vi "ResetKnob.vi"(1 "name":string, 2 "camera":u64, 3 "knobRef":refnum<vi>) -> ()   [LabVIEW 2019]
uses:
  EmergentCameraC/EmergentCameraC.lvlib
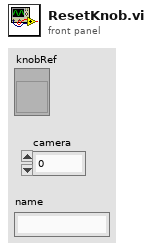
[diagram p1: front panel]
types:
  T1 = enum8{"Enabled", "Disabled", "Disabled and Grayed Out"}
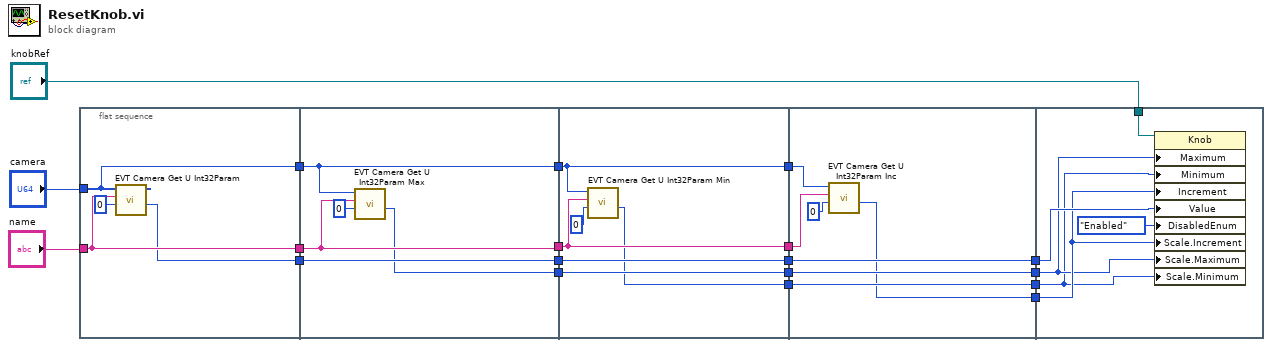
[diagram p0: block diagram]
diagram:
  n1 = flat-sequence {
    tunnel: "camera" -> [w21]
    tunnel: "name" -> [w22]
    tunnel: [w22] -> w17
    tunnel: [w21] -> w14
    tunnel: [w20] -> w7
    tunnel: w17 -> [w28]
    tunnel: [w28] -> w16
    tunnel: w14 -> [w26]
    tunnel: [w26] -> w12
    tunnel: [w25] -> w8
    tunnel: w7 -> [w25]
    tunnel: [w24] -> w4
    tunnel: w16 -> [w34]
    tunnel: [w34] -> w15
    tunnel: [w32] -> w13
    tunnel: w12 -> [w32]
    tunnel: [w31] -> w9
    tunnel: w8 -> [w31]
    tunnel: [w30] -> w5
    tunnel: w4 -> [w30]
    tunnel: [w29] -> w2
    tunnel: w15 -> [w41]
    tunnel: w13 -> [w39]
    tunnel: [w38] -> w10
    tunnel: w9 -> [w38]
    tunnel: [w37] -> w6
    tunnel: w5 -> [w37]
    tunnel: [w36] -> w3
    tunnel: w2 -> [w36]
    tunnel: [w35] -> w1
    tunnel: "knobRef" -> [w46]
    tunnel: w10 -> [w45]
    tunnel: w6 -> [w43]
    tunnel: w3 -> [w42]
    tunnel: w1 -> [w44]
    frame #0 {
      n2 = call "EVT Camera Get U Int32Param.vi"("val"=u32 0, "name"=w22, "camera"=w21) -> ("val out"=w20:u32)  [unwired: 7 in, 1 out]
    }
    frame #1 {
      n3 = call "EVT Camera Get U Int32Param Max.vi"("max"=u32 0, "name"=w28, "camera"=w26) -> ("max out"=w24:u32)  [unwired: 7 in, 1 out]
    }
    frame #2 {
      n4 = call "EVT Camera Get U Int32Param Min.vi"("min"=u32 0, "name"=w34, "camera"=w32) -> ("min out"=w29:u32)  [unwired: 7 in, 1 out]
    }
    frame #3 {
      n5 = call "EVT Camera Get U Int32Param Inc.vi"("inc"=u32 0, "name"=w41, "camera"=w39) -> ("inc out"=w35:u32)  [unwired: 7 in, 1 out]
    }
    frame #4 {
      n6 = property class="Knob"(reference=w46, "Maximum"=w43, "Minimum"=w42, "Increment"=w44, "Value"=w45, "DisabledEnum"=T1."Enabled" ("Disabled"), "Scale.Increment"=w44, "Scale.Maximum"=w43, "Scale.Minimum"=w42) -> ()  [unwired: 1 in, 2 out]
    }
  }
